vi "solar_misc Netstat Port Status.vi"(8 "error in (no error)":errorcluster, 11 "Port":u16) -> (0 "error out":errorcluster, 2 "State":T1(ring), 3 "dup Port":u16)   [LabVIEW 2018]
doc: "This checks the port status using the 'netstat' command line function."
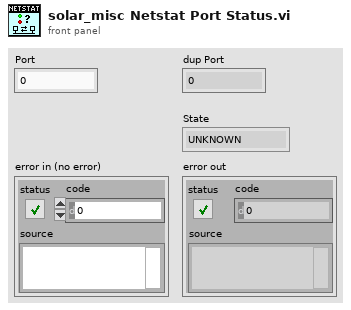
[diagram p1: front panel]
types:
  T1 = enum8{"UNKNOWN", "LISTEN", "ESTABLISHED", "SYN_SENT", "SYN_RECV", "LAST_ACK", "CLOSE_WAIT", "TIME_WAIT", "CLOSED", "CLOSING", "FIN_WAIT1", "FIN_WAIT2"}
  T2 = cluster{"Protocol":enum16{"invalid", "tcp", "udp", "icmp", "ip", "tcpv6", "udpv6", "icmpv6", "ipv6"}, "LocalIP":string, "LocalPort":u16, "ForeignIP":string, "ForeignPort":u16, "State":enum8{"UNKNOWN", "LISTEN", "ESTABLISHED", "SYN_SENT", "SYN_RECV", "LAST_ACK", "CLOSE_WAIT", "TIME_WAIT", "CLOSED", "CLOSING", "FIN_WAIT1", "FIN_WAIT2"}}[]
  T3 = cluster{"Protocol":enum16{"invalid", "tcp", "udp", "icmp", "ip", "tcpv6", "udpv6", "icmpv6", "ipv6"}, "LocalIP":string, "LocalPort":u16, "ForeignIP":string, "ForeignPort":u16, "State":enum8{"UNKNOWN", "LISTEN", "ESTABLISHED", "SYN_SENT", "SYN_RECV", "LAST_ACK", "CLOSE_WAIT", "TIME_WAIT", "CLOSED", "CLOSING", "FIN_WAIT1", "FIN_WAIT2"}}
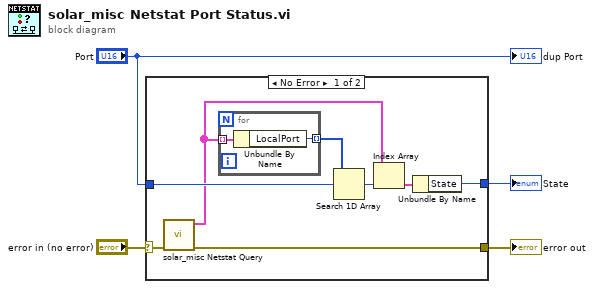
[diagram p0: block diagram]
diagram:
  n1 = case shown="No Error" "error in (no error)" {
    selector: "error in (no error)" -> [w12 w15]
    tunnel: [w11 w15] -> w3
    tunnel: "Port" -> [w9 _]
    tunnel: [w5 _] -> w2
    frame No Error {
      n2 = call "solar_misc Netstat Query.vi"("error in (no error)"=w12) -> ("error out"=w11:errorcluster, "netstat"=w7:T2)  [unwired: 9 in]
      n3 = for {
        tunnel: w7 -> [w14] mode=indexing
        tunnel: [w13] -> w10 mode=indexing
        n4 = Unbundle By Name(w14) -> ("LocalPort"=w13:u16)
      }
      n5 = Search 1D Array(1D array=w10, element=w9) -> (index of element=w8:i32)  [unwired: 1 in]
      n6 = Index Array(array=w7, index=w8) -> (element=w6:T3)
      n7 = Unbundle By Name(w6) -> ("State"=w5:T1)
    }
    frame Error {
    }
  }
  "error out" <- w3
  "State" <- w2
  "dup Port" <- "Port"
